vi "OAT Get Magnitude and Phase From Order Waveform.vi"(7 "order":dbl=1.0 format="%.2f", 8 "pulse/revolution (1)":i32=1, 9 "speed profile":T1 {"speed [RPM]" format="%.2f"; "time [s]" format="%.2f"}, 11 "order waveform [EU]":waveform(dbl)={"t0"=timestamp(0 s since 1904-01-01), "dt"=0.00025, "Y"=[]}) -> (2 "phase lag":dbl[](array[numeric]) format="%.2f", 3 "magnitudes (RMS)":dbl[](array[numeric]) format="%.2f")   [LabVIEW 2017, in "SoundVib_Resampling.lvlib"]
uses:
  <vilib>/addons/Sound and Vibration/Order Analysis/Resample Order Tracking/SoundVib_Resampling.lvlib
  <vilib>/addons/Sound and Vibration/Order Analysis/Tach Process/SubVIs/speed profile.ctl
  <vilib>/Analysis/5stat.llb/RMS (DBL).vi
  <vilib>/Analysis/NI_AALBase.lvlib
  <vilib>/Analysis/NI_AALPro.lvlib
  <vilib>/addons/Sound and Vibration/Order Analysis/Tach Process/SoundVib_TachProcess.lvlib
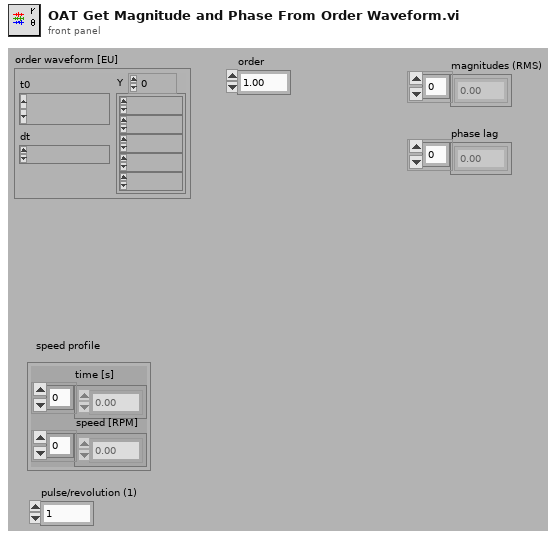
[diagram p1: front panel]
types:
  T1 = typedef "SoundVib_TachProcess.lvlib/speed profile.ctl" = cluster{"time [s]":dbl[], "speed [RPM]":dbl[]}
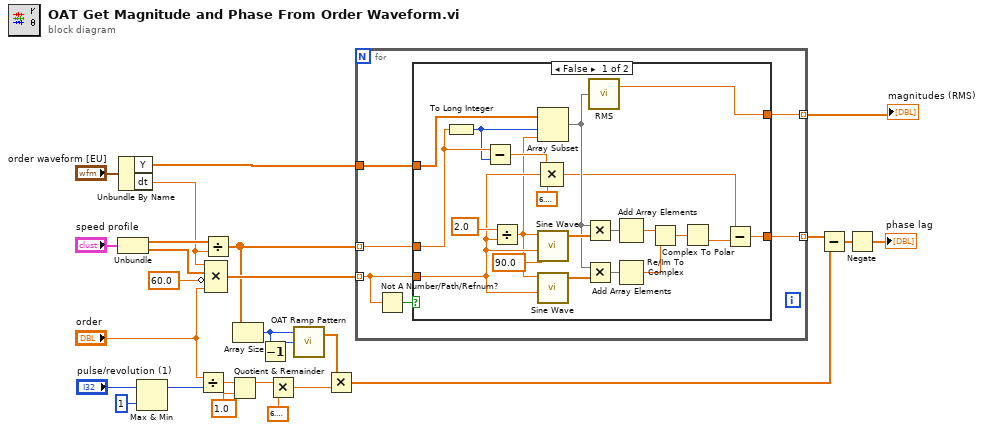
[diagram p0: block diagram]
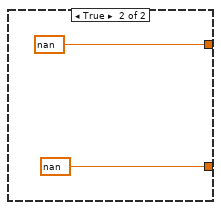
[diagram p2: hidden frame]
diagram:
  n1 = Unbundle("speed profile") -> ("time [s]"=w24:dbl[], "speed [RPM]"=w23:dbl[])
  n2 = Unbundle By Name("order waveform [EU]") -> ("Y"=w9:dbl[], "dt"=w21:dbl)
  n3 = Max & Min(x="pulse/revolution (1)", y=1) -> (max(x,y)=w3:i32)  [unwired: 1 out]
  n4 = Divide(x="order", y=w3) -> (x/y=w18:dbl)
  n5 = Divide(x=w24, y=w21) -> (x/y=w7:dbl[])
  n6 = Compound Arithmetic op=MULTIPLY(w21, w23, invert 60.0, "order") -> (w8:dbl[])
  n7 = Quotient & Remainder(x=w18, y=1.0) -> (x-y*floor(x/y)=w14:dbl)  [unwired: 1 out]
  n8 = Array Size(array=w7) -> (size(s)=w16:i32)
  n9 = Decrement(x=w16) -> (x-1=w15:i32)
  n10 = Multiply(x=w14, y=6.283185307179586) -> (x*y=w10:dbl)
  n11 = call <vilib>:"OAT Ramp Pattern.vi"("end"=w15, "samples"=w16) -> ("Ramp Pattern"=w13:dbl[])  [unwired: 1 in, 1 out]
  n12 = Multiply(x=w13, y=w10) -> (x*y=w11:dbl[])
  n13 = for {
    tunnel: w7 -> [w31] mode=indexing
    tunnel: w9 -> [w32]
    tunnel: [w29] -> w6 mode=indexing
    tunnel: w8 -> [w27] mode=indexing
    tunnel: [w30] -> w12 mode=indexing
    n14 = Not A Number/Path/Refnum?(number/path/refnum=w27) -> (NaN/Path/Refnum?=w28:bool)
    n15 = case shown="False" w28 {
      tunnel: w32 -> [w53 _]
      tunnel: w31 -> [w52 _]
      tunnel: w27 -> [w45 _]
      tunnel: [w35 nan ("rms value")] -> w30
      tunnel: [w34 nan ("rms value")] -> w29
      frame False {
        n16 = To Long Integer(number=w52) -> (32bit integer=w51:i32)
        n17 = Subtract(x=w52, y=w51) -> (x-y=w49:dbl)
        n18 = Divide(x=2.0 ("cycles"), y=w45) -> (x/y=w33:dbl)
        n19 = Array Subset(array=w53, index=w51, length=w33) -> (w43:dbl[])
        n20 = call <vilib>:"Sine Wave.vi"("samples"=w33, "frequency"=w45, "phase in"=90.0) -> ("sine wave"=w48:dbl[])  [unwired: 2 in, 2 out]
        n21 = call <vilib>:"Sine Wave.vi"("samples"=w33, "frequency"=w45) -> ("sine wave"=w44:dbl[])  [unwired: 3 in, 2 out]
        n22 = Compound Arithmetic op=MULTIPLY(w49, w45, 6.283185307179586) -> (w36:dbl)
        n23 = Multiply(x=w43, y=w48) -> (x*y=w47:dbl[])
        n24 = Multiply(x=w43, y=w44) -> (x*y=w42:dbl[])
        n25 = call-poly <vilib>:"RMS.vi"("X"=w43) -> ("rms value"=w34:dbl)  [unwired: 1 out]
        n26 = Add Array Elements(numeric array=w47) -> (sum=w41:dbl)
        n27 = Add Array Elements(numeric array=w42) -> (sum=w40:dbl)
        n28 = Re/Im To Complex(1:w40, 2:w41) -> (0:w38:cdb)
        n29 = Complex To Polar(r * e^(i*theta)=w38) -> (theta=w37:dbl)  [unwired: 1 out]
        n30 = Subtract(x=w36, y=w37) -> (x-y=w35:dbl)
      }
      frame True {
      }
    }
  }
  "magnitudes (RMS)" <- w6
  n31 = Subtract(x=w12, y=w11) -> (x-y=w5:dbl[])
  n32 = Negate(x=w5) -> (-x=→"phase lag":dbl[])
